vi "ProcessHandshakeRequest.vi"(8 "error in (no error)":errorcluster, 11 "HTTP Headers":string) -> (0 "error out":errorcluster, 1 "Sec-WebSocket-Key":string, 2 "Path":string, 3 "Is Websocket Request?":bool, 4 "Headers Out":variant, 5 "Host":string)   [LabVIEW 2013, in "WebSockets.lvlib"]
uses:
  WebSockets.lvlib
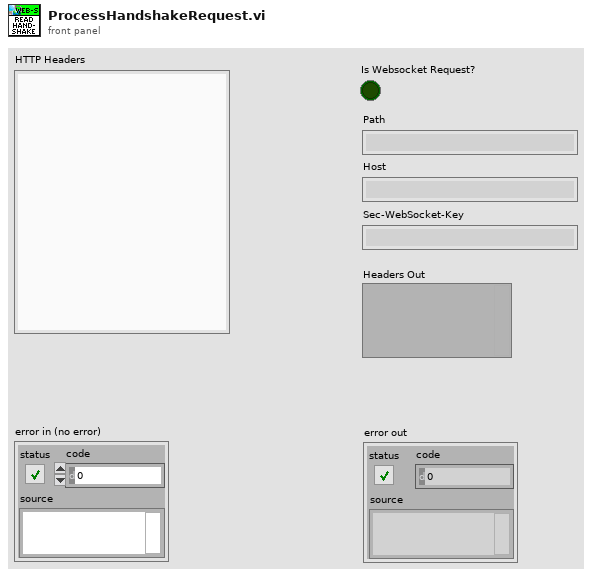
[diagram p1: front panel]
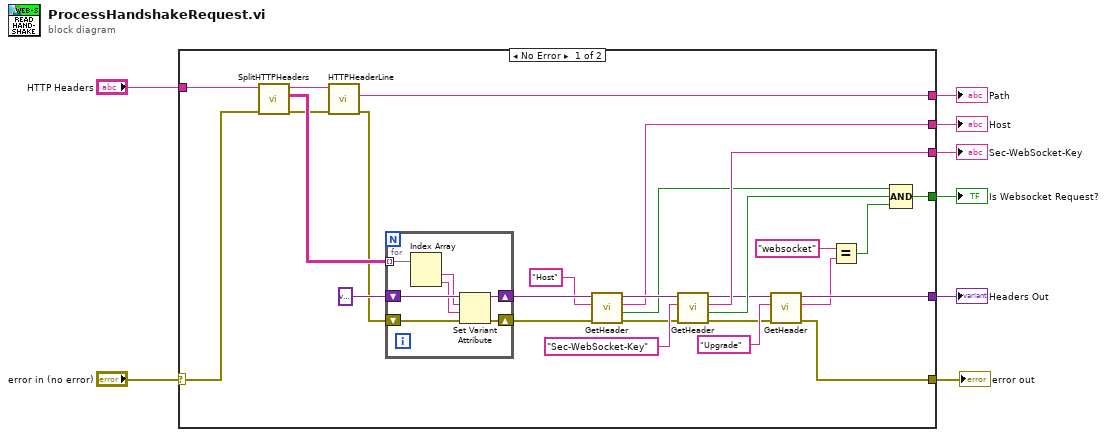
[diagram p0: block diagram]
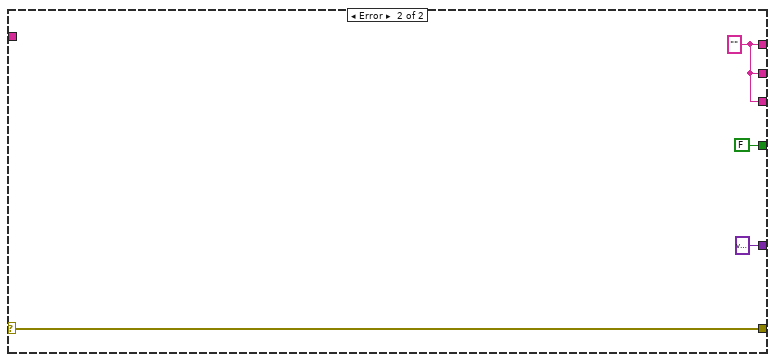
[diagram p2: hidden frame]
diagram:
  n1 = case shown="No Error" "error in (no error)" {
    selector: "error in (no error)" -> [w15 w46]
    tunnel: "HTTP Headers" -> [w35 _]
    tunnel: [w31 w44] -> w7
    tunnel: [w27 w44] -> w6
    tunnel: [w25 w44] -> w5
    tunnel: [w21 variant ("Headers Out")] -> w4
    tunnel: [w16 FALSE] -> w3
    tunnel: [w11 w46] -> w1
    frame No Error {
      n2 = call "SplitHTTPHeaders.vi"("error in (no error)"=w15, "HTTP Header String"=w35) -> ("error out"=w14:errorcluster, "Headers Array"=w33:string[][], "HTTP Request"=w34:string)  [unwired: 7 in]
      n3 = call "HTTPHeaderLine.vi"("error in (no error)"=w14, "HTTP Request Line"=w34) -> ("error out"=w9:errorcluster, "Request URI"=w31:string)  [unwired: 6 in, 2 out]
      n4 = for {
        tunnel: w33 -> [w42] mode=indexing
        shift-right: [w40] -> w30
        shift-left: variant -> [w41]
        shift-right: [w37] -> w10
        shift-left: w9 -> [w36]
        n5 = Index Array(array=w42) -> (element #1=w39:string, element #2=w38:string)  [unwired: 2 in]
        n6 = Set Variant Attribute(Variant=w41, name=w39, value=w38, error in=w36) -> (Variant out=w40:variant, error out=w37:errorcluster)  [unwired: 1 out]
      }
      n7 = call "GetHeader.vi"("error in (no error)"=w10, "Name"="Host" ("name"), "Headers In"=w30) -> ("error out"=w13:errorcluster, "Found?"=w24:bool, "Data"=w27:string, "Headers Out"=w28:variant)  [unwired: 5 in]
      n8 = call "GetHeader.vi"("error in (no error)"=w13, "Name"="Sec-WebSocket-Key", "Headers In"=w28) -> ("error out"=w12:errorcluster, "Found?"=w23:bool, "Data"=w25:string, "Headers Out"=w22:variant)  [unwired: 5 in]
      n9 = call "GetHeader.vi"("error in (no error)"=w12, "Name"="Upgrade", "Headers In"=w22) -> ("error out"=w11:errorcluster, "Data"=w19:string, "Headers Out"=w21:variant)  [unwired: 5 in, 1 out]
      n10 = Equal?(x="websocket", y=w19) -> (x = y?=w17:bool)
      n11 = Compound Arithmetic op=AND(w24, w23, w17) -> (w16:bool)
    }
    frame Error {
      w44 = "" ("Request URI")
    }
  }
  "Host" <- w6
  "Path" <- w7
  "Sec-WebSocket-Key" <- w5
  "Is Websocket Request?" <- w3
  "Headers Out" <- w4
  "error out" <- w1
